vi "RichToFlatcif_plugincore_GetNamesRequest.vi"(5 "OutputClusterType":T1, 11 "InputCluster":T2) -> (3 "OutputCluster":T1)   [LabVIEW 2021, in "CIFCorePlugin_client.lvlib"]
uses:
  CIFCorePlugin_client.lvlib
  cif_plugincore_GetNamesRequest.ctl
  cif_plugincore_GetNamesRequest_Flat.ctl
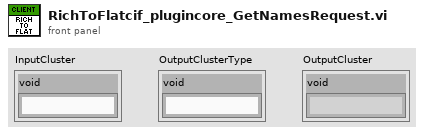
[diagram p1: front panel]
types:
  T1 = typedef "CIFCorePlugin_client.lvlib/cif_plugincore_GetNamesRequest_Flat.ctl" = cluster{"void":string}
  T2 = typedef "CIFCorePlugin_client.lvlib/cif_plugincore_GetNamesRequest.ctl" = cluster{"void":string}
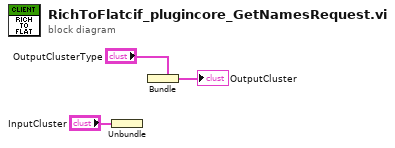
[diagram p0: block diagram]
diagram:
  n1 = Unbundle "Unbundle"("InputCluster") -> ()  [unwired: 1 out]
  n2 = Bundle "Bundle"(cluster="OutputClusterType") -> (→"OutputCluster":T1)  [unwired: 1 in]
